vi "Prepare and send data via alert (subVi).vi"(2 "error in (no error)":errorcluster, 3 "Average array":dbl[][](array[numeric]), 4 "target":string) -> (0 "error out":errorcluster, 1 "result dict":string)   [LabVIEW 2016]
uses:
  <vilib>/Distrio/LabbitMQ/Connection/Connection.lvclass
  global/Config_Infos.vi
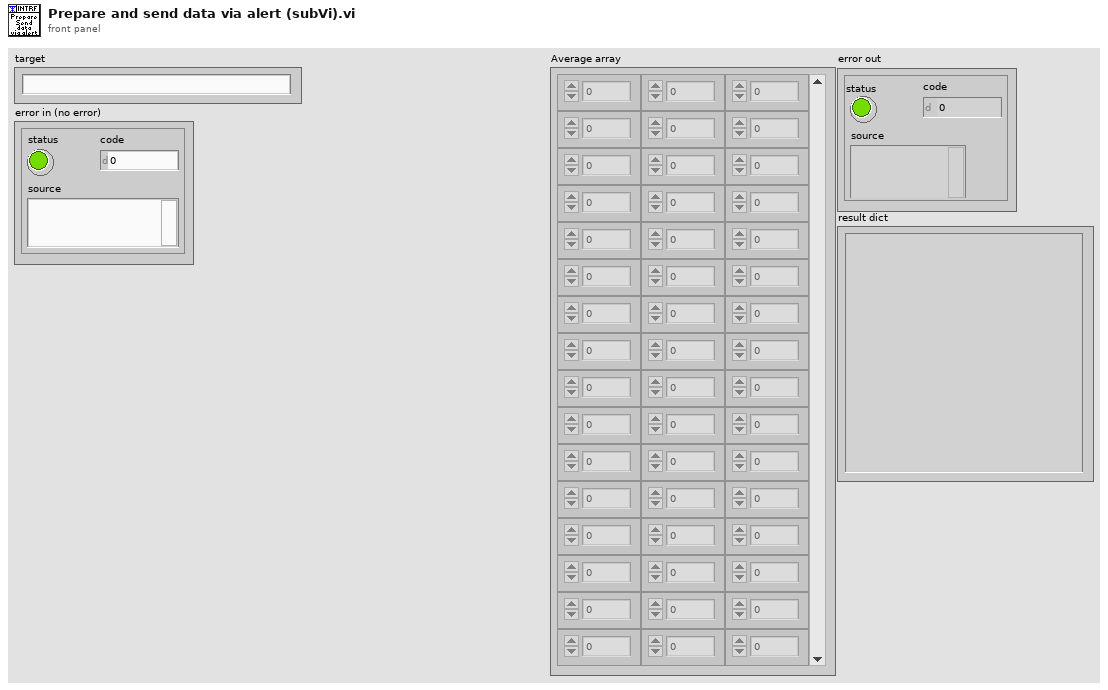
[diagram p1: front panel]
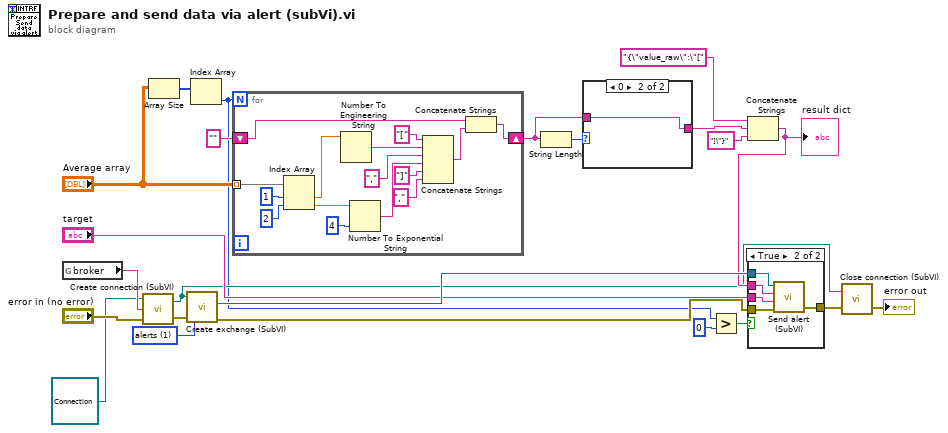
[diagram p0: block diagram]
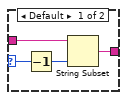
[diagram p3: hidden frame]
diagram:
  w6 = u16 1 items=["requests", "alerts"] ("exchange name")
  n1 = global read "Config_Infos.vi" "broker"() -> (w23:string)
  n2 = call "Create connection (SubVI).vi"("error in (no error)"="error in (no error)", "host name"=w23, "Connection in"=refnum<class "Connection.lvclass"> refnum) -> ("error out"=w15:errorcluster, "Connection out"=w9:refnum<class "Connection.lvclass">)
  n3 = Array Size(array="Average array") -> (size(s)=w21:i32[])
  n4 = call "Create exchange (SubVI).vi"("Connection in"=w9, "exchange name"=w6, "error in (no error)"=w15) -> ("Exchange.lvclass"=w14:refnum<class "Exchange.lvclass">, "error out"=w13:errorcluster)  [unwired: 2 out]
  n5 = Index Array(array=w21) -> (element=w3:i32)  [unwired: 1 in]
  n6 = for {
    N: w3 -> [_]
    tunnel: "Average array" -> [w38] mode=indexing
    shift-right: [w26] -> w18
    shift-left: "" -> [w27]
    n7 = Index Array(array=w38, index #1=1 ("index"), index #2=2 ("index")) -> (element #1=w33:dbl, element #2=w35:dbl)
    n8 = Number To Engineering String(4:w33) -> (0:w32:string)  [unwired: 3 in]
    n9 = Number To Exponential String(number=w35, precision (6)=i16 4) -> (E-format string=w30:string)  [unwired: 2 in]
    n10 = Concatenate Strings("[" ("string"), w32, "," ("string"), w30, "]" ("string"), "," ("string")) -> (w25:string)
    n11 = Concatenate Strings(w27, w25) -> (w26:string)
  }
  n12 = String Length(string=w18) -> (length=w19:i32)
  n13 = case shown="0" w19 {
    selector: w19 -> [w41 _]
    tunnel: w18 -> [w42 w43]
    tunnel: [w39 w43] -> w5
    frame Default {
      n14 = Decrement(x=w41) -> (x-1=w40:i32)
      n15 = String Subset(string=w42, length (rest)=w40) -> (substring=w39:string)  [unwired: 1 in]
    }
    frame 0 {
    }
  }
  n16 = Greater?(x=w3, y=0) -> (0:w4:bool)
  n17 = Concatenate Strings("{\"value_raw\":\"[" ("string"), w5, "]\"}" ("string")) -> (w12:string)
  "result dict" <- w12
  n18 = case shown="True" w4 {
    tunnel: w14 -> [_ w49]
    tunnel: w13 -> [w44 w48]
    tunnel: w12 -> [_ w47]
    tunnel: "target" -> [_ w46]
    tunnel: [w44 w45] -> w10
    frame False {
    }
    frame True {
      n19 = call "Send alert (SubVI).vi"("error in (no error)"=w48, "target"=w46, "message content"=w47, "Exchange.lvclass"=w49) -> ("error out"=w45:errorcluster)  [unwired: 2 out]
    }
  }
  n20 = call "Close connection (SubVI).vi"("error in (no error)"=w10, "Connection in"=w9) -> ("error out"=→"error out":errorcluster)  [unwired: 1 in]
